vi "CThread Schedule.vi"   [LabVIEW 2012, in "CThread.lvlib"]
uses:
  CThread.lvlib
  XNodes/terminalnode/CThread VI Terminal Node.xnode
  Core/CThread Thread Properties.ctl
  CRef/Interface/CRef Boolean.llb/Boolean CReference.ctl
  CRef/CRef.lvlib
  Base/CThread Base - Schedule Run.vi
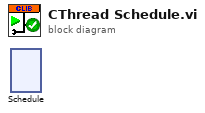
[diagram p0: block diagram]
diagram:
  n1 = xnode "Schedule"() -> ()  [unwired: 2 in, 2 out]
